vi "P1Y1.vi"() -> ()   [LabVIEW 2020]
panel:
  out "concatenated string":string
  out "x*y":dbl
  in  "x":dbl
  in  "length (rest) 2":i32
  in  "offset (0) 2":i32
  in  "offset":i32
  in  "length (rest)":i32
  in  "offset (0)":i32
  in  "string 2":string
  in  "Boolean 2":bool
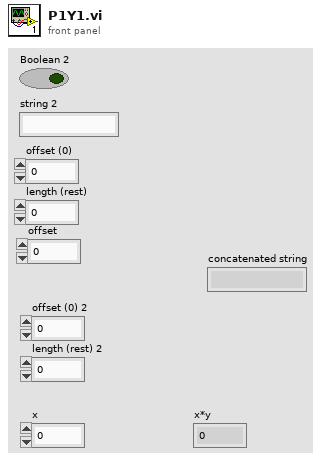
[diagram p1: front panel]
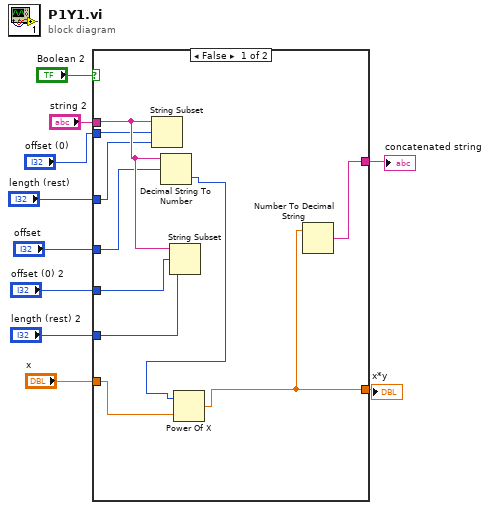
[diagram p0: block diagram]
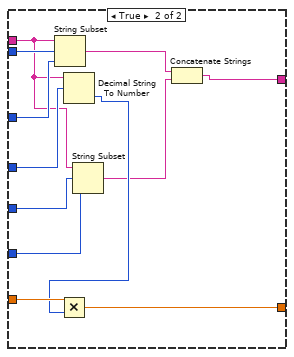
[diagram p2: hidden frame]
diagram:
  n1 = case shown="False" "Boolean 2" {
    tunnel: "string 2" -> [w20 w29]
    tunnel: "offset (0)" -> [w19 w32]
    tunnel: "length (rest)" -> [w18 w31]
    tunnel: "offset" -> [w17 w30]
    tunnel: "offset (0) 2" -> [w16 w28]
    tunnel: "length (rest) 2" -> [w15 w27]
    tunnel: "x" -> [w14 w26]
    tunnel: [w11 w24] -> w2
    tunnel: [w12 w21] -> w1
    frame False {
      n2 = String Subset(string=w20, offset (0)=w19, length (rest)=w18) -> ()  [unwired: 1 out]
      n3 = Decimal String To Number(string=w20, offset=w17) -> (number=w13:i32)  [unwired: 1 in, 1 out]
      n4 = String Subset(string=w20, offset (0)=w16, length (rest)=w15) -> ()  [unwired: 1 out]
      n5 = Power Of X(1:w14, 2:w13) -> (0:w11:dbl)
      n6 = Number To Decimal String(number=w11) -> (decimal integer string=w12:string)  [unwired: 1 in]
    }
    frame True {
      n7 = String Subset(string=w29, offset (0)=w32, length (rest)=w31) -> (substring=w23:string)
      n8 = Decimal String To Number(string=w29, offset=w30) -> (number=w25:i32)  [unwired: 1 in, 1 out]
      n9 = Multiply(x=w26, y=w25) -> (x*y=w24:dbl)
      n10 = String Subset(string=w29, offset (0)=w28, length (rest)=w27) -> (substring=w22:string)
      n11 = Concatenate Strings(w23, w22) -> (w21:string)
    }
  }
  "x*y" <- w2
  "concatenated string" <- w1
